vi "SettingManager.vi"() -> ()   [LabVIEW 2019]
uses:
  <vilib>/Utility/cursorutil.llb/Set Cursor (Icon Pict).vi
  <vilib>/regexp/Match Regular Expression.xnode
  SettingManager/SavedSettingsOptions.ctl
panel:
  in  "Tab Control":enum32{"Description", "Options"}(tab)
  in  "Description":string
  in  "Options":T1
  out "CurrentSetting":string
  out "PerviousSelection":string[](array[string])
  out "Modified":bool
  in  "Delete":bool
  in  "Restore":bool
  in  "Title":string
  in  "Save":bool
  in  "Saved Settings":string(tree)
  in  "Reload Control Tree":bool
  in  "Tree":string[](tree)
  # "<====>"
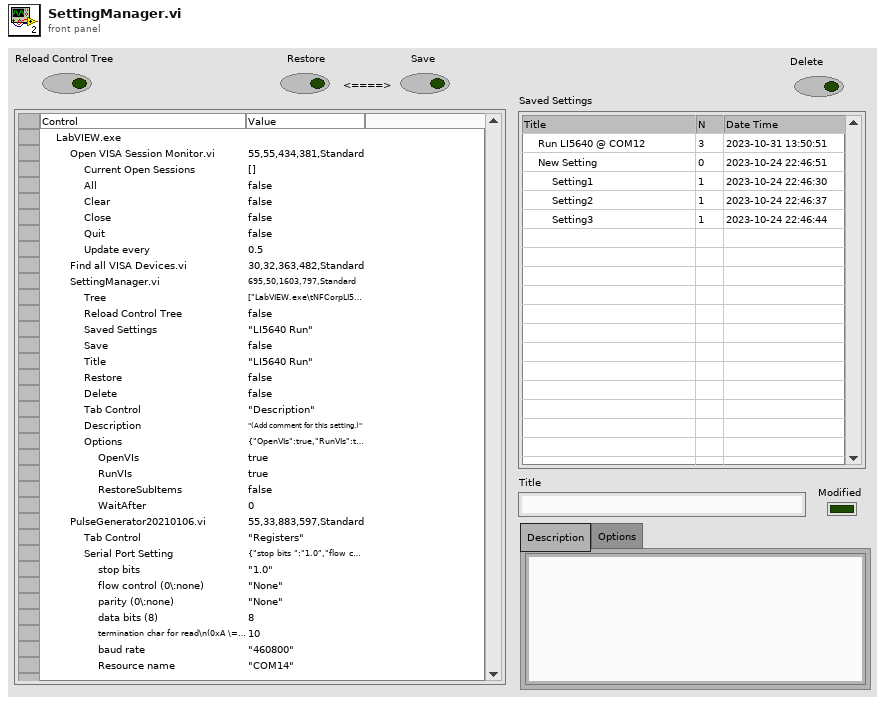
[diagram p1: front panel]
types:
  T1 = typedef "SavedSettingsOptions.ctl" = cluster{"OpenVIs":bool, "RunVIs":bool, "RestoreSubItems":bool, "WaitAfter":u32}
  T2 = cluster{"Name":string, "Include Shift Key?":bool, "Include Ctrl Key?":bool, "Shortcut Key":string}[]
  T3 = cluster{"Closed Nodes":string[], "Selection":string[], "Defer Panel Update":bool}
  T4 = enum16{"Left Button", "Center Button", "Right Button", "Window Close"}
  T5 = typedef "eventvkey.ctl" = enum16{"ASCII", "Enter", "Return", "Shift", "Ctrl", "Alt", "Cmd", "Opt", "Caps", "NumLock", "Clear", "Break", "Up", "Down", "Left", "Right", "Insert", "Delete", "Home", "End", "PageUp", "PageDown", "Escape", "Help", "Pause", "ScrollLock", "F1", "F2", "F3", "F4", "F5", "F6", "F7", "F8", "F9", "F10", "F11", "F12", "F13", "F14", "F15", "F16", "F17", "F18", "F19", "F20", "F21", "F22", "F23", "F24", "Play", "VolumeUp", "VolumeDown", "Mute", "Two Byte Char"}
  T6 = typedef "LVPoint32TypeDef.ctl" = cluster{"Horizontal":i32, "Vertical":i32}
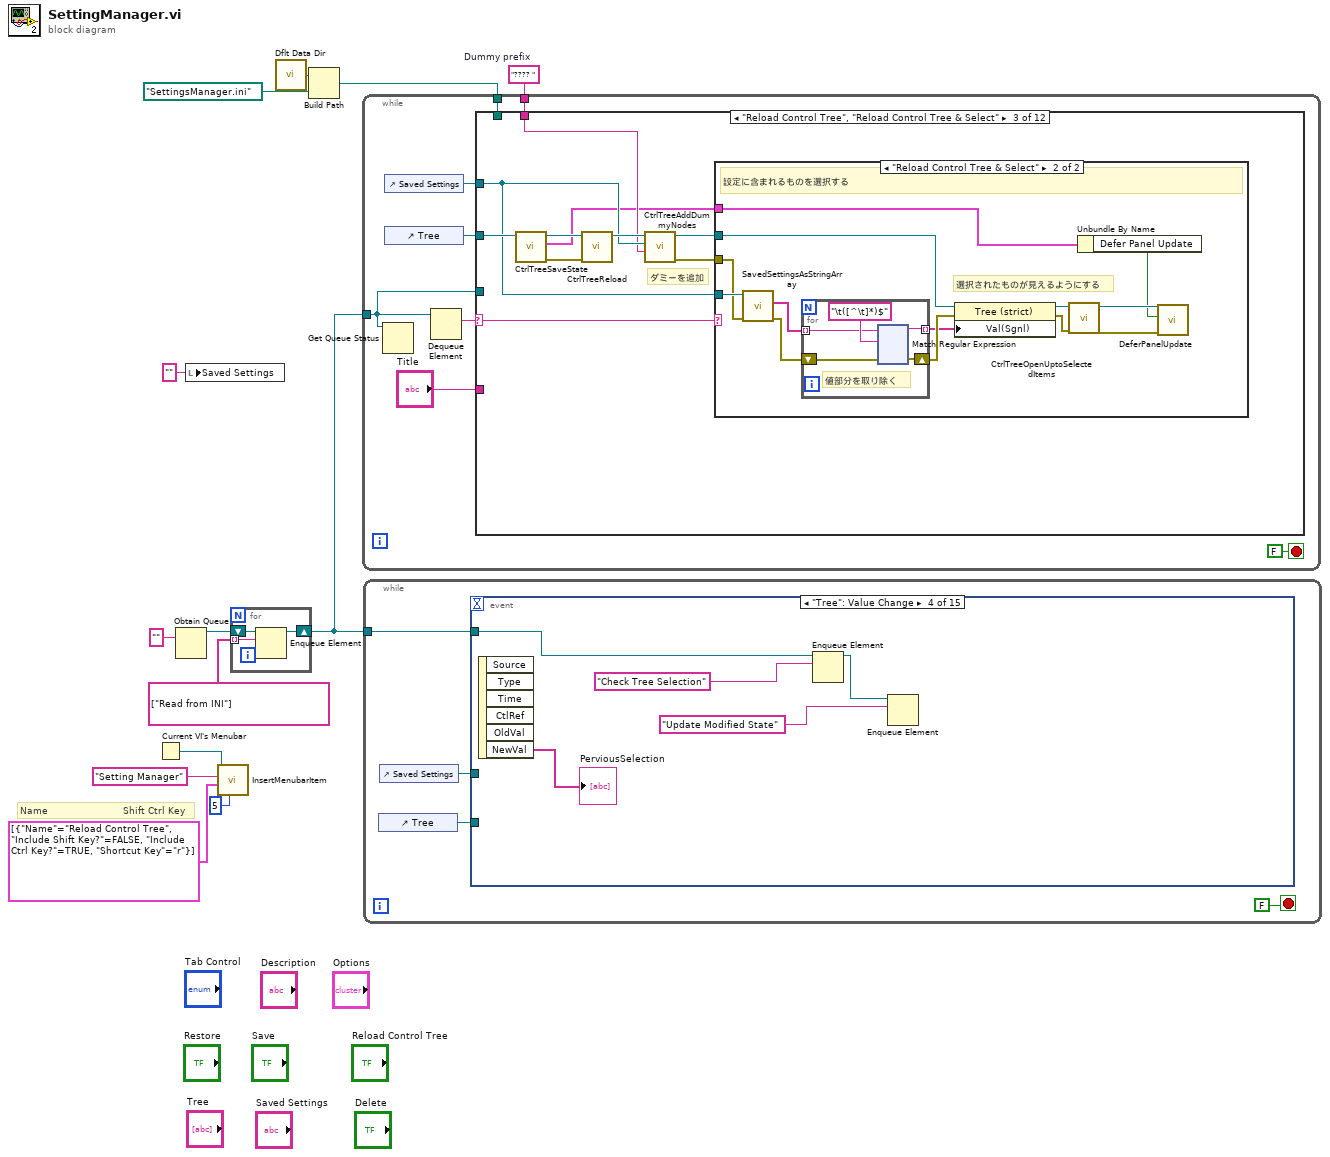
[diagram p0: block diagram]
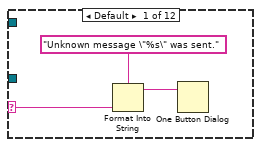
[diagram p2: hidden frame]
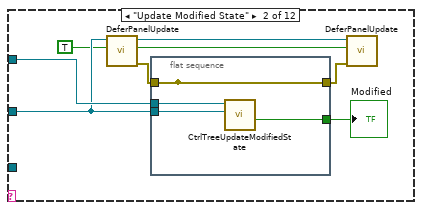
[diagram p3: hidden frame]
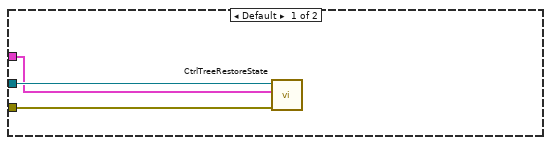
[diagram p4: hidden frame]
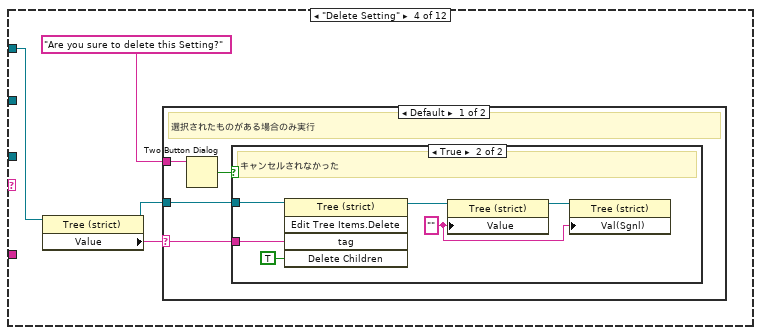
[diagram p5: hidden frame]
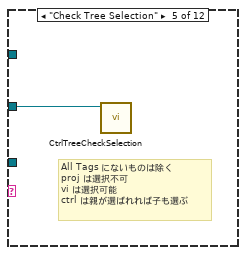
[diagram p8: hidden frame]
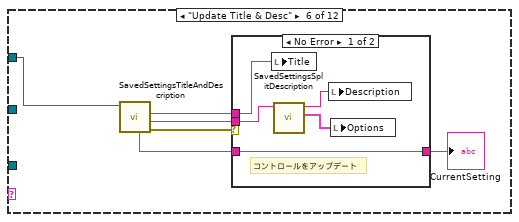
[diagram p9: hidden frame]
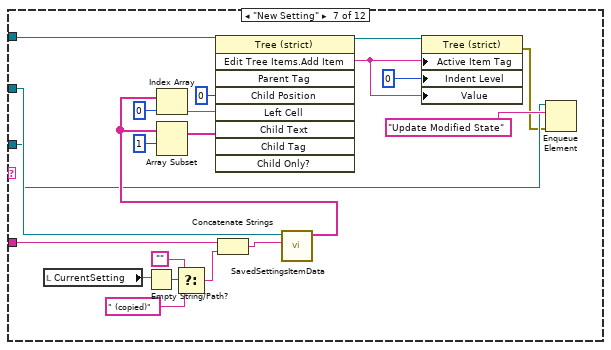
[diagram p11: hidden frame]
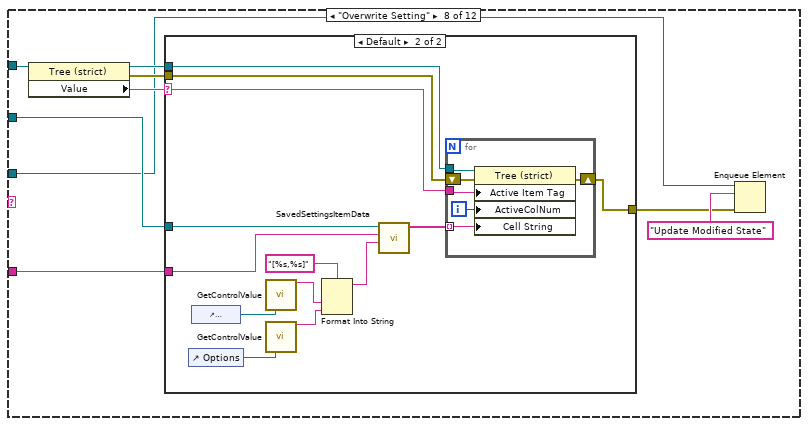
[diagram p12: hidden frame]
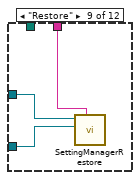
[diagram p14: hidden frame]
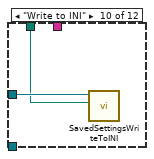
[diagram p15: hidden frame]
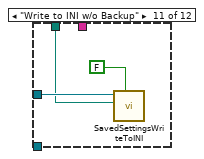
[diagram p16: hidden frame]
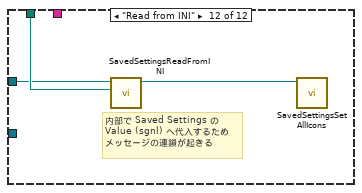
[diagram p17: hidden frame]
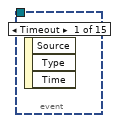
[diagram p18: hidden frame]
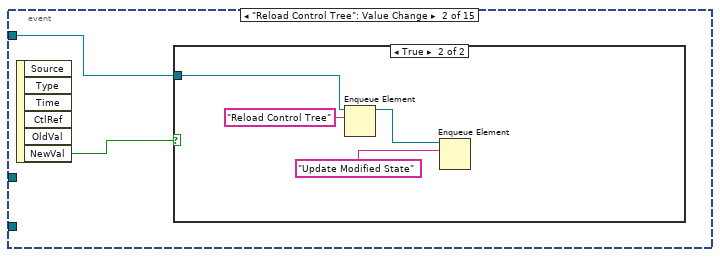
[diagram p19: hidden frame]
diagram:
  w10 = "???? "  # Dummy prefix
  # "Name                         Shift Ctrl Key"
  n1 = Current VI's Menubar() -> (w4:refnum<k9>)
  n2 = Obtain Queue(element data type="") -> (queue out=w12:refnum<queue>)  [unwired: 4 in, 2 out]
  n3 = local write "Saved Settings"("" ("Saved Settings")) -> ()
  n4 = call "InsertMenubarItem.vi"("Insert After (last)"=5, "Sub Items"=T2 [{"Name"="Reload Control Tree", "Include Shift Key?"=FALSE, "Include Ctrl Key?"=TRUE, "Shortcut Key"="r"}] ("Menu Short Cut"), "Menu Name"="Setting Manager", "menu ref"=w4) -> ()  [unwired: 3 in, 5 out]
  n5 = for {
    tunnel: string[] ["Read from INI"] ("element") -> [w15] mode=indexing
    shift-right: [w14] -> w11
    shift-left: w12 -> [w16]
    n6 = Enqueue Element(queue=w16, element=w15) -> (queue out=w14:refnum<queue>)  [unwired: 2 in, 2 out]
  }
  n7 = call <vilib>:"Dflt Data Dir.vi"() -> ("App:Default Data Directory"=w7:path)
  n8 = Build Path(base path=w7, name or relative path=path "SettingsManager.ini" ("default name")) -> (appended path=w8:path)
  n9 = while {
    tunnel: w11 -> [w17]
    tunnel: w10 -> [w19]
    tunnel: w8 -> [w18]
    stop <- FALSE stop-if-true
    n10 = Get Queue Status(queue=w17) -> ()  [unwired: 2 in, 8 out]
    n11 = control-ref of="Saved Settings"() -> (w21:refnum<vi>)
    n12 = control-ref of="Tree"() -> (w22:refnum<vi>)
    n13 = Dequeue Element(queue=w17) -> (element=w24:string)  [unwired: 2 in, 3 out]
    n14 = case shown="\"Reload Control Tree\", \"Reload Control Tree & Select\"" w24 {
      selector: w24 -> [w26 _ w48 _ _ _ _ _ _ _ _ _]
      tunnel: w22 -> [_ w33 w49 _ w202 _ w232 w243 w265 _ _ _]
      tunnel: w21 -> [_ w35 w44 w189 _ w205 w234 w241 w266 w268 w271 w273]
      tunnel: "Title" -> [_ _ _ _ _ _ w229 w242 _ _ _ _]
      tunnel: w17 -> [_ _ _ _ _ _ w222 w235 _ _ _ _]
      tunnel: w19 -> [_ _ w43 _ _ _ _ _ w264 _ _ _]
      tunnel: w18 -> [_ _ _ _ _ _ _ _ _ w267 w270 w274]
      frame Default {
        n15 = Format Into String(format string="Unknown message \"%s\" was sent.", w26) -> (resulting string=w25:string)  [unwired: 2 in, 1 out]
        n16 = One Button Dialog(message=w25) -> ()  [unwired: 1 in, 1 out]
      }
      frame "Update Modified State" {
        n17 = call "DeferPanelUpdate.vi"("Defer Panel Updates (T)"=TRUE, "Control in"=w33) -> ("error out"=w31:errorcluster, "Defer Panel Updates Old"=w29:bool, "Control out"=w32:refnum<vi>)  [unwired: 7 in]
        n18 = flat-sequence {
          tunnel: w35 -> [w39]
          tunnel: [w38] -> w34
          tunnel: w33 -> [w37]
          tunnel: w31 -> [w36]
          tunnel: [w36] -> _
          tunnel: [w36] -> w30
          frame #0 {
            n19 = call "CtrlTreeUpdateModifiedState.vi"("ControlTree in"=w37, "SavedSettings in"=w39) -> ("Boolean"=w38:bool)  [unwired: 9 in]
          }
        }
        n20 = call "DeferPanelUpdate.vi"("error in (no error)"=w30, "Defer Panel Updates (T)"=w29, "Control in"=w32) -> ()  [unwired: 6 in, 3 out]
        "Modified" <- w34
      }
      frame "Reload Control Tree", "Reload Control Tree & Select" {
        # "ダミーを追加"
        n21 = call "CtrlTreeSaveState.vi"("TreeControl in"=w49) -> ("error out"=w42:errorcluster, "State"=w40:T3, "TreeControl out"=w47:refnum<vi>)  [unwired: 8 in]
        n22 = call "CtrlTreeReload.vi"("error in (no error)"=w42, "TreeControl in"=w47) -> ("TreeControl out"=w46:refnum<vi>)  [unwired: 9 in]
        n23 = call "CtrlTreeAddDummyNodes.vi"("Dummy prefix"=w43, "SavedSettings in"=w44, "TreeControl in"=w46) -> ("error out"=w41:errorcluster, "TreeControl out"=w45:refnum<vi>)  [unwired: 7 in]
        n24 = case shown="\"Reload Control Tree & Select\"" w48 {
          tunnel: w45 -> [w51 w63]
          tunnel: w44 -> [_ w64]
          tunnel: w41 -> [w52 w61]
          tunnel: w40 -> [w50 w56]
          frame Default {
            n25 = call "CtrlTreeRestoreState.vi"("error in (no error)"=w52, "State"=w50, "TreeControl in"=w51) -> ()  [unwired: 7 in, 2 out]
          }
          frame "Reload Control Tree & Select" {
            # "選択されたものが見えるようにする"
            # "設定に含まれるものを選択する"
            n26 = call "SavedSettingsAsStringArray.vi"("error in (no error)"=w61, "SavedSettings in"=w64) -> ("error out"=w60:errorcluster, "Selection"=w65:string[])  [unwired: 5 in, 3 out]
            n27 = for {
              tunnel: w65 -> [w69] mode=indexing
              tunnel: [w68] -> w57 mode=indexing
              shift-right: [w66] -> w59
              shift-left: w60 -> [w67]
              # "値部分を取り除く"
              n28 = xnode "Match Regular Expression"("input string"=w69, "regular expression"="\t([^\t]*)$", "error in"=w67) -> ("before match"=w68:string, "error out"=w66:errorcluster)  [unwired: 3 in, 3 out]
            }
            n29 = property class="Tree (strict)"(reference=w63, error in=w59, "Val(Sgnl)"=w57) -> (reference out=w62:refnum<vi>, error out=w58:errorcluster)
            n30 = call "CtrlTreeOpenUptoSelectedItems.vi"("error in (no error)"=w58, "TreeControl in"=w62) -> ("error out"=w54:errorcluster, "TreeControl out"=w55:refnum<vi>)  [unwired: 8 in]
            n31 = Unbundle By Name(w56) -> ("Defer Panel Update"=w53:bool)
            n32 = call "DeferPanelUpdate.vi"("error in (no error)"=w54, "Defer Panel Updates (T)"=w53, "Control in"=w55) -> ()  [unwired: 6 in, 3 out]
          }
        }
      }
      frame "Delete Setting" {
        n33 = property class="Tree (strict)"(reference=w189) -> (reference out=w191:refnum<vi>, "Value"=w188:string)  [unwired: 1 in, 1 out]
        n34 = case shown="Default" w188 {
          selector: w188 -> [w192 _]
          tunnel: "Are you sure to delete this Setting?" ("message") -> [w195 _]
          tunnel: w191 -> [w193 _]
          frame Default {
            # "選択されたものがある場合のみ実行"
            n35 = Two Button Dialog(message=w195) -> (T button?=w194:bool)  [unwired: 2 in]
            n36 = case shown="True" w194 {
              tunnel: w192 -> [_ w201]
              tunnel: w193 -> [_ w199]
              frame False {
              }
              frame True {
                w196 = "" ("Active Item:Tag")
                # "キャンセルされなかった"
                n37 = invoke class="Tree (strict)" method="Edit Tree Items.Delete"(reference=w199, "tag"=w201, "Delete Children"=TRUE ("Delete Children?")) -> (reference out=w198:refnum<vi>)  [unwired: 2 in, 4 out]
                n38 = property class="Tree (strict)"(reference=w198, "Value"=w196) -> (reference out=w197:refnum<vi>)  [unwired: 1 in, 1 out]
                n39 = property class="Tree (strict)"(reference=w197, "Val(Sgnl)"=w196) -> ()  [unwired: 1 in, 2 out]
              }
            }
          }
          frame "" {
          }
        }
      }
      frame "Check Tree Selection" {
        # "All Tags にないものは除く\nproj は選択不可\nvi は選択可能\nctrl は親が選ばれれば子も選ぶ"
        n40 = call "CtrlTreeCheckSelection.vi"("TreeControl in"=w202) -> ()  [unwired: 9 in, 2 out]
      }
      frame "Update Title & Desc" {
        n41 = call "SavedSettingsTitleAndDescription.vi"("TreeControl in"=w205) -> ("error out"=w208:errorcluster, "Description"=w207:string, "Title"=w206:string, "Value"=w204:string)  [unwired: 6 in, 1 out]
        n42 = case shown="No Error" w208 {
          tunnel: w206 -> [w213 _]
          tunnel: w207 -> [w212 _]
          tunnel: w204 -> [w211 _]
          tunnel: [w211 _] -> w203
          frame No Error {
            # "コントロールをアップデート"
            n43 = local write "Title"(w213) -> ()
            n44 = call "SavedSettingsSplitDescription.vi"("Description in"=w212) -> ("Options"=w209:T1, "Description out"=w210:string)  [unwired: 9 in]
            n45 = local write "Description"(w210) -> ()
            n46 = local write "Options"(w209) -> ()
          }
          frame Error {
          }
        }
        "CurrentSetting" <- w203
      }
      frame "New Setting" {
        n47 = local read "CurrentSetting"() -> (w220:string)
        n48 = Empty String/Path?(string/path=w220) -> (empty?=w219:bool)
        n49 = Select(t="", s=w219, f=" (copied)") -> (s? t:f=w215:string)
        n50 = Concatenate Strings(w229, w215) -> (w216:string)
        n51 = call "SavedSettingsItemData.vi"("Title"=w216, "CtrlTree in"=w232) -> ("Data to be saved"=w227:string[])  [unwired: 7 in, 2 out]
        n52 = Index Array(array=w227, index=0) -> (element=w224:string)
        n53 = Array Subset(array=w227, index=1) -> (w225:string[])  [unwired: 1 in]
        n54 = invoke class="Tree (strict)" method="Edit Tree Items.Add Item"(reference=w234, "Child Position"=0, "Left Cell"=w224, "Child Text"=w225) -> (reference out=w231:refnum<vi>, "Edit Tree Items:Add Item"=w221:string)  [unwired: 5 in, 7 out]
        n55 = property class="Tree (strict)"(reference=w231, "Active Item Tag"=w221, "Indent Level"=0 ("Active Item:Indent Level"), "Value"=w221) -> (error out=w214:errorcluster)  [unwired: 1 in, 1 out]
        n56 = Enqueue Element(queue=w222, element="Update Modified State", error in (no error)=w214) -> ()  [unwired: 1 in, 3 out]
      }
      frame "Overwrite Setting" {
        n57 = property class="Tree (strict)"(reference=w241) -> (reference out=w239:refnum<vi>, error out=w237:errorcluster, "Value"=w240:string)  [unwired: 1 in]
        n58 = case shown="Default" w240 {
          selector: w240 -> [_ w255]
          tunnel: w243 -> [_ w257]
          tunnel: w242 -> [_ w256]
          tunnel: w239 -> [_ w253]
          tunnel: w237 -> [w244 w252]
          tunnel: [w244 w251] -> w236
          frame "" {
          }
          frame Default {
            n59 = control-ref of="Options"() -> (w249:refnum<vi>)
            n60 = control-ref of="Description"() -> (w250:refnum<vi>)
            n61 = call "GetControlValue.vi"("control ref"=w250) -> ("String out"=w248:string)  [unwired: 12 in, 2 out]
            n62 = call "GetControlValue.vi"("control ref"=w249) -> ("String out"=w247:string)  [unwired: 12 in, 2 out]
            n63 = Format Into String(format string="[%s,%s]", w248, w247) -> (resulting string=w245:string)  [unwired: 2 in, 1 out]
            n64 = call "SavedSettingsItemData.vi"("Description"=w245, "Title"=w256, "CtrlTree in"=w257) -> ("Data to be saved"=w254:string[])  [unwired: 6 in, 2 out]
            n65 = for {
              tunnel: w253 -> [w263]
              tunnel: w255 -> [w262]
              tunnel: w254 -> [w260] mode=indexing
              shift-right: [w258] -> w251
              shift-left: w252 -> [w259]
              i -> [w261]
              n66 = property class="Tree (strict)"(reference=w263, error in=w259, "Active Item Tag"=w262, "ActiveColNum"=w261, "Cell String"=w260) -> (error out=w258:errorcluster)  [unwired: 1 out]
            }
          }
        }
        n67 = Enqueue Element(queue=w235, element="Update Modified State", error in (no error)=w236) -> ()  [unwired: 1 in, 3 out]
      }
      frame "Restore" {
        n68 = call "SettingManagerRestore.vi"("Dummy prefix"=w264, "Control Tree"=w265, "Saved Settings"=w266) -> ()  [unwired: 8 in, 1 out]
      }
      frame "Write to INI" {
        n69 = call "SavedSettingsWriteToINI.vi"("Inifile path"=w267, "TreeControl in"=w268) -> ()  [unwired: 10 in]
      }
      frame "Write to INI w/o Backup" {
        n70 = call "SavedSettingsWriteToINI.vi"("Backup"=FALSE, "Inifile path"=w270, "TreeControl in"=w271) -> ()  [unwired: 9 in]
      }
      frame "Read from INI" {
        # "内部で Saved Settings の\nValue (sgnl) へ代入するため\nメッセージの連鎖が起きる"
        n71 = call "SavedSettingsReadFromINI.vi"("Inifile path"=w274, "SavedSettings in"=w273) -> ("SavedSettings out"=w272:refnum<vi>)  [unwired: 9 in]
        n72 = call "SavedSettingsSetAllIcons.vi"("TreeControl in"=w272) -> ()  [unwired: 11 in]
      }
    }
  }
  n73 = while {
    tunnel: w11 -> [w277]
    stop <- FALSE stop-if-true
    n74 = control-ref of="Tree"() -> (w275:refnum<vi>)
    n75 = control-ref of="Saved Settings"() -> (w276:refnum<vi>)
    n76 = event shown="[3] \"Tree\": Value Change" {
      selector: _ -> [_ _ _ _ _ _ _ _ _ _ _ _ _ _ _]
      dyn-events: _ -> [_ _ _ _ _ _ _ _ _ _ _ _ _ _ _]
      timeout: _ -> [_ _ _ _ _ _ _ _ _ _ _ _ _ _ _]
      tunnel: w277 -> [_ w279 w285 w295 w297 w322 w340 w346 _ _ w367 _ w390 w419 w420]
      tunnel: w276 -> [_ _ _ _ w296 _ _ _ w354 w356 _ _ w391 _ _]
      tunnel: w275 -> [_ _ _ _ _ w317 _ _ _ _ _ w385 w389 _ _]
      event Timeout {
        n77 = event-data() -> ()  [unwired: 1 in, 3 out]
      }
      event "Reload Control Tree": Value Change {
        n78 = event-data() -> ("NewVal"=w280:bool)  [unwired: 1 in, 5 out]
        n79 = case shown="True" w280 {
          tunnel: w279 -> [_ w284]
          frame False {
          }
          frame True {
            n80 = Enqueue Element(queue=w284, element="Reload Control Tree") -> (queue out=w281:refnum<queue>)  [unwired: 2 in, 2 out]
            n81 = Enqueue Element(queue=w281, element="Update Modified State") -> ()  [unwired: 2 in, 3 out]
          }
        }
      }
      event Menu Selection (User) {
        n82 = event-data() -> ("ItemTag"=w286:string)  [unwired: 1 in, 6 out]
        n83 = case shown="\"Reload Control Tree\"" w286 {
          tunnel: w285 -> [_ w287]
          frame "False", Default {
          }
          frame "Reload Control Tree" {
            n84 = Enqueue Element(queue=w287, element="Reload Control Tree") -> (queue out=w288:refnum<queue>)  [unwired: 2 in, 2 out]
            n85 = Enqueue Element(queue=w288, element="Update Modified State") -> ()  [unwired: 2 in, 3 out]
          }
        }
      }
      event "Tree": Value Change {
        n86 = event-data() -> ("NewVal"=→"PerviousSelection":string[])  [unwired: 1 in, 5 out]
        n87 = Enqueue Element(queue=w295, element="Check Tree Selection") -> (queue out=w292:refnum<queue>)  [unwired: 2 in, 2 out]
        n88 = Enqueue Element(queue=w292, element="Update Modified State") -> ()  [unwired: 2 in, 3 out]
      }
      event "Save": Value Change {
        n89 = event-data() -> ("NewVal"=w298:bool)  [unwired: 1 in, 5 out]
        n90 = case shown="True" w298 {
          tunnel: w297 -> [_ w299]
          tunnel: w296 -> [_ w302]
          frame False {
          }
          frame True {
            n91 = property class="Tree (strict)"(reference=w302) -> ("Value"=w301:string)  [unwired: 1 in, 2 out]
            n92 = case shown="Default" w301 {
              tunnel: [w311 T4."Left Button" ("Which Button?")] -> w300
              frame Default {
                n93 = call <vilib>:"Three Button Dialog.vi"("Window Title (\"\")"="Save Setting" ("Window Title (\"\")"), "Center Button Text (\"No\")"="Overwrite" ("Center Button Text (\"No\")"), "Left Button Text (\"Yes\")"="Create New" ("Left Button Text (\"Yes\")"), "message"="To which setting the current values to be seved?") -> ("Which Button?"=w311:T4)  [unwired: 7 in]
              }
              frame "" {
              }
            }
            n94 = case shown="\"Center Button\"" w300 {
              tunnel: w299 -> [w304 w308 _]
              frame "Left Button" {
                # "Create New"
                n95 = for {
                  tunnel: w304 -> [w306]
                  tunnel: string[] ["Reload Control Tree", "New Setting", "Write to INI", "Update Title & Desc"] ("element") -> [w305] mode=indexing
                  n96 = Enqueue Element(queue=w306, element=w305) -> ()  [unwired: 2 in, 3 out]
                }
              }
              frame "Center Button" {
                # "Overwrite"
                n97 = for {
                  tunnel: w308 -> [w310]
                  tunnel: string[] ["Reload Control Tree", "Overwrite Setting", "Write to INI", "Update Title & Desc"] ("element") -> [w309] mode=indexing
                  n98 = Enqueue Element(queue=w310, element=w309) -> ()  [unwired: 2 in, 3 out]
                }
              }
              frame Default {
              }
            }
          }
        }
      }
      event "Saved Settings": Value Change {
        # "変更されているか調べ、\nキャンセルするかを尋ねる"
        n99 = event-data() -> ("CtlRef"=w321:refnum<vi>, "OldVal"=w318:string, "NewVal"=w320:string)  [unwired: 1 in, 3 out]
        n100 = case shown="Default" w318 {
          selector: w318 -> [w332 w335]
          tunnel: [w334 FALSE ("Boolean")] -> w324
          tunnel: w321 -> [w333 _]
          tunnel: [w332 w335] -> w319
          tunnel: w317 -> [w331 _]
          frame Default {
            n101 = call "CtrlTreeUpdateModifiedState.vi"("Selection"=w332, "ControlTree in"=w331, "SavedSettings in"=w333) -> ("Boolean"=w334:bool)  [unwired: 8 in]
          }
          frame "" {
          }
        }
        n102 = case shown="True" w324 {
          tunnel: w321 -> [_ _]
          tunnel: [TRUE w338] -> w323
          frame False {
          }
          frame True {
            n103 = Two Button Dialog(message="Control selection was changed. Are you sure to discard it?") -> (T button?=w338:bool)  [unwired: 2 in]
          }
        }
        n104 = case shown="True" w323 {
          tunnel: w322 -> [_ w328]
          tunnel: w321 -> [w326 _]
          tunnel: w320 -> [_ _]
          tunnel: w319 -> [w325 _]
          frame False {
            # "元に戻す"
            # "元に戻す"
            n105 = property class="Tree (strict)"(reference=w326, "Value"=w325) -> ()  [unwired: 1 in, 2 out]
          }
          frame True {
            # "選択が変更された"
            n106 = for {
              tunnel: w328 -> [w330]
              tunnel: string[] ["Update Title & Desc", "Reload Control Tree & Select", "Write to INI w/o Backup"] ("element") -> [w329] mode=indexing
              n107 = Enqueue Element(queue=w330, element=w329) -> ()  [unwired: 2 in, 3 out]
            }
          }
        }
      }
      event "Restore": Value Change {
        n108 = event-data() -> ("NewVal"=w341:bool)  [unwired: 1 in, 5 out]
        n109 = case shown="True" w341 {
          tunnel: w340 -> [_ w343]
          frame False {
          }
          frame True {
            n110 = for {
              tunnel: string[] ["Reload Control Tree", "Update Modified State", "Restore", "Reload Control Tree"] -> [w345] mode=indexing
              tunnel: w343 -> [w344]
              n111 = Enqueue Element(queue=w344, element=w345) -> ()  [unwired: 2 in, 3 out]
            }
          }
        }
      }
      event "Saved Settings": Key Down {
        n112 = event-data() -> ("VKey"=w347:T5)  [unwired: 1 in, 9 out]
        n113 = case shown="\"Delete\"" w347 {
          tunnel: w346 -> [_ w348]
          frame Default {
          }
          frame "Delete" {
            n114 = for {
              tunnel: w348 -> [w351]
              tunnel: string[] ["Delete Setting", "Write to INI"] ("element") -> [w350] mode=indexing
              n115 = Enqueue Element(queue=w351, element=w350) -> ()  [unwired: 2 in, 3 out]
            }
          }
        }
      }
      event "Title": Value Change {
        w353 = u16 0 items=["Title"=0, "Description"=3] ("Witch")
        n116 = event-data() -> ("NewVal"=w355:string)  [unwired: 1 in, 5 out]
        n117 = local read "CurrentSetting"() -> (w352:string)
        n118 = call "SavedSettingsSetTitleOrDescription.vi"("Witch"=w353, "Value"=w355, "Tag"=w352, "TreeControl in"=w354) -> ()  [unwired: 6 in, 2 out]
      }
      event "Description": Value Change {
        w366 = u16 3 items=["Title"=0, "Description"=3] ("Witch")
        n119 = event-data() -> ()  [unwired: 1 in, 6 out]
        n120 = local read "CurrentSetting"() -> (w357:string)
        n121 = control-ref of="Description"() -> (w365:refnum<vi>)
        n122 = control-ref of="Options"() -> (w364:refnum<vi>)
        n123 = call "GetControlValue.vi"("control ref"=w365) -> ("String out"=w362:string)  [unwired: 12 in, 2 out]
        n124 = call "GetControlValue.vi"("control ref"=w364) -> ("String out"=w363:string)  [unwired: 12 in, 2 out]
        n125 = local read "Options"() -> (w359:T1)
        n126 = Format Into String(format string="[%s,%s]", w362, w363) -> (resulting string=w360:string)  [unwired: 2 in, 1 out]
        n127 = Unbundle By Name(w359) -> ("RestoreSubItems"=w358:bool)
        n128 = call "SavedSettingsSetTitleOrDescription.vi"("Witch"=w366, "Value"=w360, "Tag"=w357, "TreeControl in"=w356) -> ()  [unwired: 6 in, 2 out]
        n129 = call "SavedSettingsSetIcon.vi"("Restore SubItems"=w358, "Tag"=w357, "TreeControl in"=w356) -> ()  [unwired: 7 in, 2 out]
      }
      event "Delete": Value Change {
        n130 = event-data() -> ("NewVal"=w368:bool)  [unwired: 1 in, 5 out]
        n131 = case shown="True" w368 {
          tunnel: w367 -> [_ w371]
          frame False {
          }
          frame True {
            n132 = for {
              tunnel: w371 -> [w373]
              tunnel: string[] ["Delete Setting", "Write to INI"] ("element") -> [w372] mode=indexing
              n133 = Enqueue Element(queue=w373, element=w372) -> ()  [unwired: 2 in, 3 out]
            }
            n134 = local write "Delete"(FALSE ("Delete")) -> ()
          }
        }
      }
      event "Tree": Mouse Move {
        n135 = event-data() -> ("Coords"=w384:T6)  [unwired: 1 in, 4 out]
        n136 = invoke class="Tree (strict)" method="Point To Row Column"(reference=w385, "Point"=w384) -> (reference out=w383:refnum<vi>, error out=w382:errorcluster, "Tag"=w381:string, "InGlyph"=w376:bool)  [unwired: 6 in, 4 out]
        n137 = property class="Tree (strict)"(reference=w383, error in=w382, "Active Item Tag"=w381) -> (error out=w378:errorcluster, "Indent Level"=w380:i32)  [unwired: 1 out]
        n138 = Unbundle By Name(w378) -> ("status"=w374:bool)
        n139 = Equal?(x=w380, y=1) -> (x = y?=w375:bool)
        n140 = Compound Arithmetic op=AND(invert w374, w375, w376) -> (w377:bool)
        n141 = case shown="False" w377 {
          frame False {
            n142 = call-poly <vilib>:"Set Cursor.vi"("icon"=u16 1) -> ()  [unwired: 9 in, 2 out]
          }
          frame True {
            n143 = call-poly <vilib>:"Set Cursor.vi"("icon"=u16 6) -> ()  [unwired: 9 in, 2 out]
          }
        }
      }
      event "Tree": Mouse Down {
        n144 = event-data() -> ("Coords"=w402:T6)  [unwired: 1 in, 7 out]
        n145 = local read "PerviousSelection"() -> (w388:string[])
        n146 = invoke class="Tree (strict)" method="Point To Row Column"(reference=w389, "Point"=w402) -> (reference out=w401:refnum<vi>, error out=w400:errorcluster, "Tag"=w392:string, "InGlyph"=w395:bool)  [unwired: 6 in, 4 out]
        n147 = property class="Tree (strict)"(reference=w401, error in=w400, "Active Item Tag"=w392) -> (error out=w397:errorcluster, "Indent Level"=w399:i32)  [unwired: 1 out]
        n148 = Equal?(x=w399, y=1) -> (x = y?=w394:bool)
        n149 = Unbundle By Name(w397) -> ("status"=w393:bool)
        n150 = Compound Arithmetic op=AND(invert w393, w394, w395) -> (w396:bool)
        n151 = case shown="True" w396 {
          tunnel: w389 -> [_ w403]
          tunnel: w392 -> [_ w414]
          tunnel: w391 -> [_ w413]
          tunnel: w390 -> [_ w412]
          tunnel: w388 -> [_ w405]
          frame False {
          }
          frame True {
            n152 = call "SavedSettingsAppsAndVIs.vi"("SavedSettings in"=w413) -> ("VIs"=w406:map{string, string}, "Apps"=w407:map{string, string})  [unwired: 7 in, 2 out]
            n153 = call "CtrlTreeOpenVI.vi"("VIs"=w406, "Apps"=w407, "Tag"=w414, "ControlTree in"=w403) -> ("error out"=w409:errorcluster, "Newly Opened"=w411:bool, "VI ref"=w408:refnum<vi>)  [unwired: 5 in]
            n154 = invoke class="VI" method="FP.Open"(reference=w408, error in=w409, "Activate"=TRUE ("Activate?")) -> (error out=w404:errorcluster)  [unwired: 2 in, 4 out]
            n155 = property class="Tree (strict)"(reference=w403, error in=w404, "Val(Sgnl)"=w405) -> ()  [unwired: 2 out]
            n156 = case shown="True" w411 {
              tunnel: w412 -> [_ w416]
              frame False {
              }
              frame True {
                n157 = Enqueue Element(queue=w416, element="Reload Control Tree") -> ()  [unwired: 2 in, 3 out]
              }
            }
          }
        }
      }
      event "Saved Settings": Drag Ended; "Saved Settings": Item Close; "Saved Settings": event #0x1e {
        n158 = event-data() -> ("CtlRef"=w417:refnum<vi>)  [unwired: 1 in, 3 out]
        n159 = call "SavedSettingsSetAllIcons.vi"("TreeControl in"=w417) -> ()  [unwired: 11 in]
        n160 = Enqueue Element(queue=w419, element="Write to INI w/o Backup") -> ()  [unwired: 2 in, 3 out]
      }
      event "Saved Settings": Double Click {
        n161 = event-data() -> ("Tag"=w421:string)  [unwired: 1 in, 9 out]
        n162 = case shown="Default" w421 {
          tunnel: w420 -> [w422 _]
          frame Default {
            n163 = for {
              tunnel: string[] ["Reload Control Tree", "Update Modified State", "Restore", "Reload Control Tree"] -> [w425] mode=indexing
              tunnel: w422 -> [w424]
              n164 = Enqueue Element(queue=w424, element=w425) -> ()  [unwired: 2 in, 3 out]
            }
          }
          frame "" {
          }
        }
      }
    }
  }
